vi "3458A Self Calibrate Virtual Channels.vi"(8 "error in":errorcluster, 10 "Ignore GUI, force selfcal (False)":bool, 11 "digitizer session in":T1={"channels"=[], "sync unit"={"VISA"="", "type"=enum."Picotest U6200A"}, "awg unit"={"type"=enum."Agilent 331xxA to 332xxA", "VISA"="", "enable 10MHz ref"=FALSE, "cmi ckd2"={"VISA"="", "clock source"=enum."Auto", "manual ref clk"=FALSE, "ref clock [Hz]"=0.0, "div mode"=enum."Set divisor directly"}, "cmi sync v3"={"VISA"="", "baud rate [bd/s]"=115200, "source"=enum."Auto", "hv range"=enum."1kV", "fsrc is fixed"=FALSE, "fsrc [Hz]"=10000000.0, "freq integ [s]"=1.0, "freq filter"=5, "trig level"=enum."TTL 5V", "chn1 mode"=enum."Source divider", "chn1 level"=enum."Positive 5V", "chn2 mode"=enum."Source divider", "chn2 level"=enum."Positive 5V", "chn2 div"=1, "chn3 mode"=enum."Chn 1 Active", "chn3 level"=enum."Positive 5V", "chn1 div entry"=enum."Calculate nearest divisor from measured fx", "chn1 dev limit [%]"=1.0, "chn1 check dev"=FALSE}, "trigger"={"source"=enum."Immediate", "level [V]"=0.0, "coupling"=enum."DC", "slope"=enum."POS"}}, "sync mode"=enum."MASTER-SLAVE, MASTER clocked by TIMER", "streaming mode"=FALSE, "idn mode"=enum."Auto", "sampling mode"=enum."DCV", "sample memory [B]"=0, "proc setup"={"channel id"=0, "packet size [smpl]"=0, "current timeout [s]"=0.0, "blk2blk timeout [s]"=0.0, "event time"=timestamp(0 s since 1904-01-01), "stop notifier"=refnum, "data queues"=[], "proc refs"=[], "bus semaphore"=refnum}, "sample size [B]"=0, "sample count"=0, "aux data"={"channel id"=0, "valid?"=[], "gain [V]"=[], "timestamp [s]"=[], "Ts [s]"=0.0, "abs timestamp"=timestamp(0 s since 1904-01-01), "t [deg C]"=[], "multiplex timestamp [s]"=-1.0, "only multiplex?"=FALSE, "multiplex smpl offset"=0, "overflow?"=FALSE}, "ranges [V]"=[], "aperture [s]"=0.0, "LEVEL trigger"={"edge"=enum."POS", "level [V]"=0.0, "coupling"=enum."DC"}, "trigger mode"=enum."AUTO", "measure temp.?"=FALSE, "disp mesages"=[], "shared bus?"=FALSE, "disable display?"=FALSE, "aper mode"=enum."Manual", "aper rules"=[], "multiplex"={"cycles"=0, "delay [s]"=0.0, "enabled"=FALSE, "overhead [s]"=1.0, "tot smpls"=0, "sub-rec"=0, "overhead [%]"=0.0, "emulated"=FALSE}, "F8588 lpf"=enum."Off", "F8588 pll"=enum."Off", "F8588 couple"=enum."DC, auto", "fs"={"freq mode"=enum."fs or Ts", "fs [Hz]"=0.0, "fref [Hz]"=0.0, "mul"=0.0, "div"=0.0}} {"awg unit"."cmi sync v3"."chn2 div" min=1 max=100000000 step=1; "awg unit"."cmi sync v3"."fsrc [Hz]" format="%_8p"; "channels"."Range [Vpk]" min=0.0}) -> (0 "error":errorcluster, 3 "digitizer session out":T1={"channels"=[], "sync unit"={"VISA"="", "type"=enum."Picotest U6200A"}, "awg unit"={"type"=enum."Agilent 331xxA to 332xxA", "VISA"="", "enable 10MHz ref"=FALSE, "cmi ckd2"={"VISA"="", "clock source"=enum."Auto", "manual ref clk"=FALSE, "ref clock [Hz]"=0.0, "div mode"=enum."Set divisor directly"}, "cmi sync v3"={"VISA"="", "baud rate [bd/s]"=115200, "source"=enum."Auto", "hv range"=enum."1kV", "fsrc is fixed"=FALSE, "fsrc [Hz]"=10000000.0, "freq integ [s]"=1.0, "freq filter"=5, "trig level"=enum."TTL 5V", "chn1 mode"=enum."Source divider", "chn1 level"=enum."Positive 5V", "chn2 mode"=enum."Source divider", "chn2 level"=enum."Positive 5V", "chn2 div"=1, "chn3 mode"=enum."Chn 1 Active", "chn3 level"=enum."Positive 5V", "chn1 div entry"=enum."Calculate nearest divisor from measured fx", "chn1 dev limit [%]"=1.0, "chn1 check dev"=FALSE}, "trigger"={"source"=enum."Immediate", "level [V]"=0.0, "coupling"=enum."DC", "slope"=enum."POS"}}, "sync mode"=enum."MASTER-SLAVE, MASTER clocked by TIMER", "streaming mode"=FALSE, "idn mode"=enum."Auto", "sampling mode"=enum."DCV", "sample memory [B]"=0, "proc setup"={"channel id"=0, "packet size [smpl]"=0, "current timeout [s]"=0.0, "blk2blk timeout [s]"=0.0, "event time"=timestamp(0 s since 1904-01-01), "stop notifier"=refnum, "data queues"=[], "proc refs"=[], "bus semaphore"=refnum}, "sample size [B]"=0, "sample count"=0, "aux data"={"channel id"=0, "valid?"=[], "gain [V]"=[], "timestamp [s]"=[], "Ts [s]"=0.0, "abs timestamp"=timestamp(0 s since 1904-01-01), "t [deg C]"=[], "multiplex timestamp [s]"=-1.0, "only multiplex?"=FALSE, "multiplex smpl offset"=0, "overflow?"=FALSE}, "ranges [V]"=[], "aperture [s]"=0.0, "LEVEL trigger"={"edge"=enum."POS", "level [V]"=0.0, "coupling"=enum."DC"}, "trigger mode"=enum."AUTO", "measure temp.?"=FALSE, "disp mesages"=[], "shared bus?"=FALSE, "disable display?"=FALSE, "aper mode"=enum."Manual", "aper rules"=[], "multiplex"={"cycles"=0, "delay [s]"=0.0, "enabled"=FALSE, "overhead [s]"=1.0, "tot smpls"=0, "sub-rec"=0, "overhead [%]"=0.0, "emulated"=FALSE}, "F8588 lpf"=enum."Off", "F8588 pll"=enum."Off", "F8588 couple"=enum."DC, auto", "fs"={"freq mode"=enum."fs or Ts", "fs [Hz]"=0.0, "fref [Hz]"=0.0, "mul"=0.0, "div"=0.0}} {"awg unit"."cmi sync v3"."chn2 div" min=1 max=100000000 step=1; "awg unit"."cmi sync v3"."fsrc [Hz]" format="%_8p"; "channels"."Range [Vpk]" min=0.0})   [LabVIEW 2020, in "3458A Virtual Digitizer.lvlib"]
doc: "This VI will allow user to initiate AUTOCAL function on all virtual channels. It will perform DCV calibartion and when the DSDC or DSAC mode is selected it will also perform ACV calibration.\nOptional input 'Ignore GUI' will perform selfcal immediately ignoring GUI buttons, then will close the panel."
uses:
  3458A Virtual Digitizer.lvlib
  3458A Digitizer Session.ctl
  3458A Virtual Channel Config.ctl
  Counter/Counter Session.ctl
  Counter/Counter Type.ctl
  AWG/AWG Session.ctl
  AWG/AWG Type.ctl
  AWG/CMI Clock Divider v2/CMI ckd2 Session.ctl
  AWG/CMI Clock Divider v2/CMI ckd2 Source Mode.ctl
  AWG/CMI Clock Divider v2/CMI ckd2 Divisor Mode.ctl
  AWG/CMI Sync V3/CMI Sync V3 session.ctl
  AWG/CMI Sync V3/Configure/CMI Sync V3 Reference Clock Source.ctl
  AWG/CMI Sync V3/Configure/CMI Sync V3 HV input Range.ctl
  AWG/CMI Sync V3/Configure/CMI Sync V3 Trigger Input Level.ctl
  AWG/CMI Sync V3/Configure/CMI Sync V3 Channel 1 Mode.ctl
  AWG/CMI Sync V3/Configure/CMI Sync V3 Channel Output Levels.ctl
  AWG/CMI Sync V3/Configure/CMI Sync V3 Channel 2 Mode.ctl
  AWG/CMI Sync V3/Configure/CMI Sync V3 Channel 3 Mode.ctl
  AWG/CMI Sync V3/Configure/CMI Sync V3 Channel 1 Divisor Entry Mode.ctl
  adc/ADC Trig Config.ctl
  adc/ADC Trig Mode Source.ctl
  adc/ADC Trig Coupling.ctl
  adc/ADC Trig Slope.ctl
  3458A Sync Mode.ctl
  3458A Idn Mode.ctl
  3458A Digitizing Low Levels/Configure/Sampling Mode.ctl
  3458A Digitizing Process Options.ctl
  3458A Data Packet.ctl
  3458A Aux Record Data.ctl
  3458A Digitizing Low Levels/Configure/Level Setup.ctl
  3458A Digitizing Low Levels/Configure/First Sample Trigger.ctl
  3458A Aperture Selection Mode.ctl
  3458A Multiplexing Config.ctl
  Fluke 8588A/F8588A Low Pass Filter.ctl
  Fluke 8588A/F8588A Phase Lock.ctl
  Fluke 8588A/F8588A Coupling.ctl
  3458A Sampling Rate.ctl
  AWG/AWG Clock Setup Mode.ctl
  3458A Digitizing Low Levels/Action-Status/AutoCal Mode.ctl
  3458A Digitizing Low Levels/3458A Digitizing Low Levels.lvlib
  3458A Basic Driver/3458A Basic Driver.lvlib
  Counter/Counter.lvlib
  AWG/AWG.lvlib
  AWG/CMI Sync V3/CMI Sync Unit V3.lvlib
panel:
  out "instructions":string="1) Disconnect everything from inputs of the DMMs. \n2) Press start to start AUTOCAL.\n3) When done, leave by EXIT.\n4) If it goes wrong, use ABORT to terminate."
  in  "btn abort":bool
  in  "btn exit":bool
  in  "btn start":bool
  out "Status":string
  out "state":i32
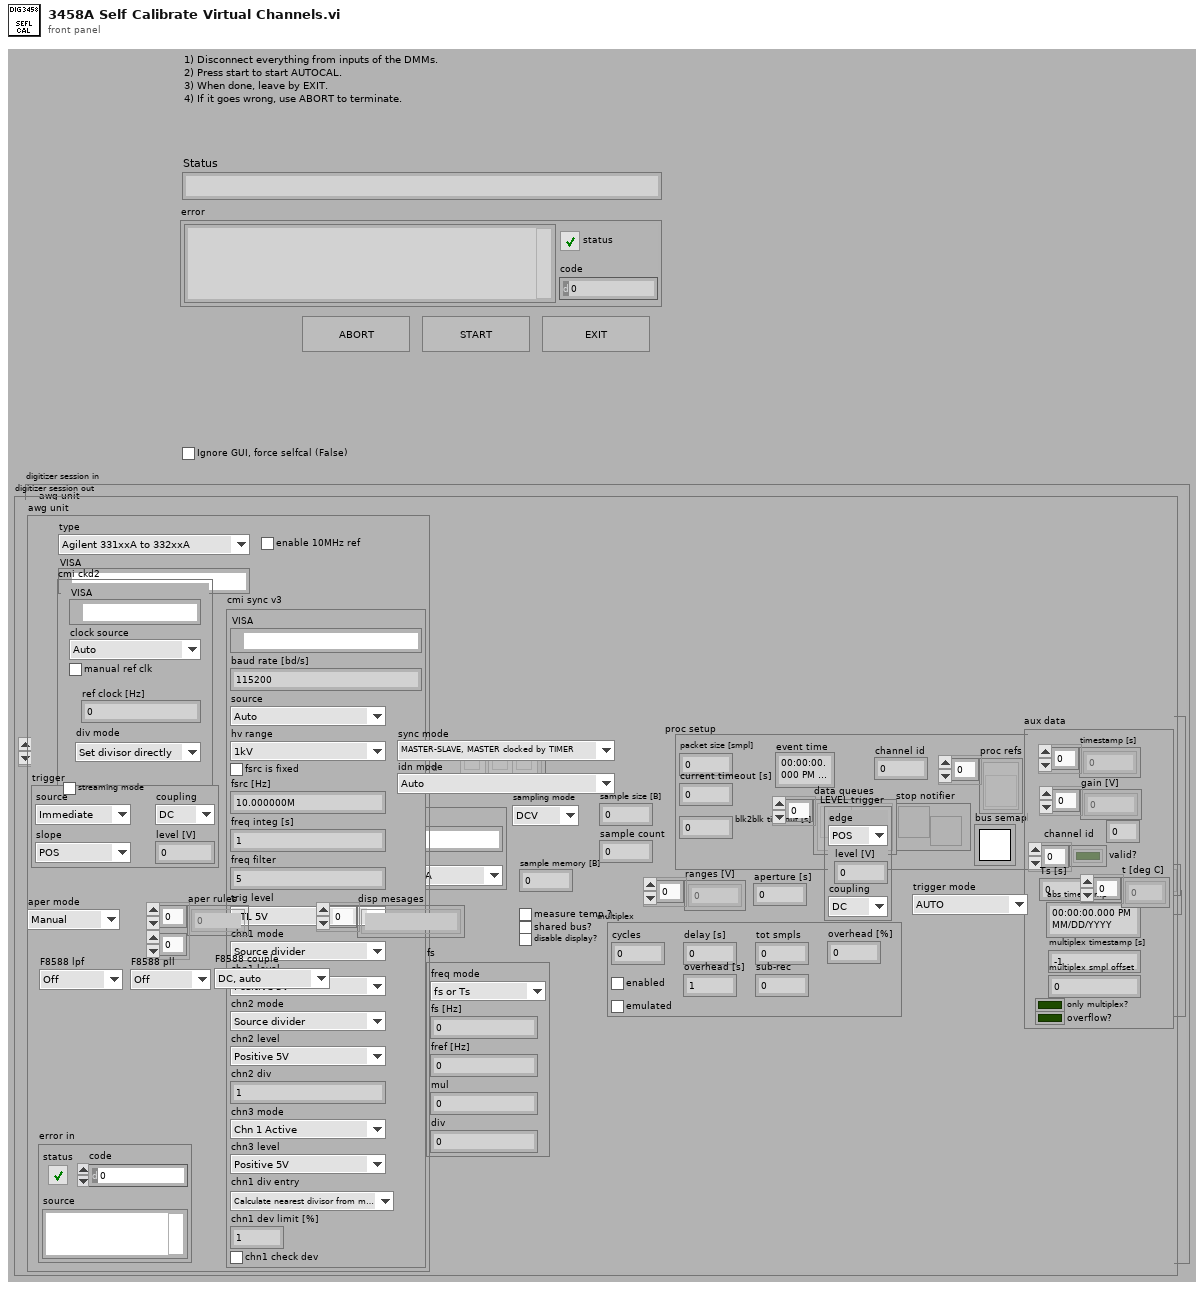
[diagram p1: front panel]
types:
  T1 = typedef "3458A Virtual Digitizer.lvlib/3458A Digitizer Session.ctl" = cluster{"channels":T2[], "sync unit":T3, "awg unit":T5, "sync mode":T23, "streaming mode":bool, "idn mode":T24, "sampling mode":T25, "sample memory [B]":i32, "proc setup":T26, "sample size [B]":i32, "sample count":i32, "aux data":T28, "ranges [V]":dbl[], "aperture [s]":dbl, "LEVEL trigger":T29, "trigger mode":T30, "measure temp.?":bool, "disp mesages":string[], "shared bus?":bool, "disable display?":bool, "aper mode":T31, "aper rules":dbl[][], "multiplex":T32, "F8588 lpf":T33, "F8588 pll":T34, "F8588 couple":T35, "fs":T36}
  T2 = typedef "3458A Virtual Digitizer.lvlib/3458A Virtual Channel Config.ctl" = cluster{"VISA":refnum<visa-resource-name>, "Range [Vpk]":dbl, "btn clr":bool, "btn up":bool, "btn down":bool, "F8588":bool, "F8588 guard":bool}
  T3 = typedef "Counter.lvlib/Counter Session.ctl" = cluster{"VISA":refnum<visa-resource-name>, "type":T4}
  T4 = typedef "Counter.lvlib/Counter Type.ctl" = enum16{"Picotest U6200A", "dummy"}
  T5 = typedef "AWG.lvlib/AWG Session.ctl" = cluster{"type":T6, "VISA":refnum<visa-resource-name>, "enable 10MHz ref":bool, "cmi ckd2":T7, "cmi sync v3":T10, "trigger":T19}
  T6 = typedef "AWG.lvlib/AWG Type.ctl" = enum16{"Agilent 331xxA to 332xxA", "Agilent 335xxA to 336xxA", "Tektronix AFG3101C", "CMI Clock Divider v2", "CMI Sync Unit V3", "dummy"}
  T7 = typedef "AWG.lvlib/CMI ckd2 Session.ctl" = cluster{"VISA":refnum<visa-resource-name>, "clock source":T8, "manual ref clk":bool, "ref clock [Hz]":dbl, "div mode":T9}
  T8 = typedef "AWG.lvlib/CMI ckd2 Source Mode.ctl" = enum16{"Auto", "LF clock", "HF clock", "Internal"}
  T9 = typedef "AWG.lvlib/CMI ckd2 Divisor Mode.ctl" = enum16{"Set divisor directly", "Set divisor by frequency"}
  T10 = typedef "AWG.lvlib/CMI Sync Unit V3.lvlib/CMI Sync V3 session.ctl" = cluster{"VISA":refnum<visa-resource-name>, "baud rate [bd/s]":i32, "source":T11, "hv range":T12, "fsrc is fixed":bool, "fsrc [Hz]":dbl, "freq integ [s]":dbl, "freq filter":i32, "trig level":T13, "chn1 mode":T14, "chn1 level":T15, "chn2 mode":T16, "chn2 level":T15, "chn2 div":i32, "chn3 mode":T17, "chn3 level":T15, "chn1 div entry":T18, "chn1 dev limit [%]":dbl, "chn1 check dev":bool}
  T11 = typedef "AWG.lvlib/CMI Sync Unit V3.lvlib/CMI Sync V3 Reference Clock Source.ctl" = enum16{"Auto", "Internal", "Logic", "Sine", "HV"}
  T12 = typedef "AWG.lvlib/CMI Sync Unit V3.lvlib/CMI Sync V3 HV input Range.ctl" = enum16{"10V", "60V", "250V", "1kV"}
  T13 = typedef "AWG.lvlib/CMI Sync Unit V3.lvlib/CMI Sync V3 Trigger Input Level.ctl" = enum16{"LVCMOS 3V3", "TTL 5V"}
  T14 = typedef "AWG.lvlib/CMI Sync Unit V3.lvlib/CMI Sync V3 Channel 1 Mode.ctl" = enum16{"Source divider", "DDS absolute", "DDS ratio", "DDS ratio M/N"}
  T15 = typedef "AWG.lvlib/CMI Sync Unit V3.lvlib/CMI Sync V3 Channel Output Levels.ctl" = enum16{"Positive 3V3", "Negative 3V3", "Positive 5V", "Negative 5V"}
  T16 = typedef "AWG.lvlib/CMI Sync Unit V3.lvlib/CMI Sync V3 Channel 2 Mode.ctl" = enum16{"Source divider", "Chn 1 divide"}
  T17 = typedef "AWG.lvlib/CMI Sync Unit V3.lvlib/CMI Sync V3 Channel 3 Mode.ctl" = enum16{"Chn 1 Active", "Chn 2 Active", "Chn 1 Trigger", "Chn 2 Trigger", "Gate", "PPS", "10MHz"}
  T18 = typedef "AWG.lvlib/CMI Sync Unit V3.lvlib/CMI Sync V3 Channel 1 Divisor Entry Mode.ctl" = enum16{"Set divisor directly", "Calculate nearest divisor from measured fx"}
  T19 = typedef "ADC Trig Config.ctl" = cluster{"source":T20, "level [V]":dbl, "coupling":T21, "slope":T22}
  T20 = typedef "ADC Trig Mode Source.ctl" = enum16{"Immediate", "External", "Level"}
  T21 = typedef "ADC Trig Coupling.ctl" = enum16{"DC", "AC"}
  T22 = typedef "ADC Trig Slope.ctl" = enum16{"POS", "NEG"}
  T23 = typedef "3458A Virtual Digitizer.lvlib/3458A Sync Mode.ctl" = enum16{"MASTER-SLAVE, MASTER clocked by TIMER", "MASTER-SLAVE, MASTER clocked by AWG", "ALL clocked by AWG", "MASTER-SLAVE, ALL clocked by TIMER", "ALL clocked by AWG with DFLL"}
  T24 = typedef "3458A Virtual Digitizer.lvlib/3458A Idn Mode.ctl" = enum16{"Auto", "Sequential (chn A, chn B, ...)", "From calibration string"}
  T25 = typedef "3458A Virtual Digitizer.lvlib/3458A Digitizing Low Levels.lvlib/Sampling Mode.ctl" = enum16{"DCV", "DSDC", "DSAC"}
  T26 = typedef "3458A Virtual Digitizer.lvlib/3458A Digitizing Process Options.ctl" = cluster{"channel id":i32, "packet size [smpl]":i32, "current timeout [s]":dbl, "blk2blk timeout [s]":dbl, "event time":timestamp, "stop notifier":refnum<notifier>, "data queues":refnum<queue>[], "proc refs":refnum<vi>[], "bus semaphore":T27}
  T27 = typedef "Semaphore RefNum" = refnum<k1>
  T28 = typedef "3458A Virtual Digitizer.lvlib/3458A Aux Record Data.ctl" = cluster{"channel id":i32, "valid?":bool[], "gain [V]":dbl[], "timestamp [s]":dbl[], "Ts [s]":dbl, "abs timestamp":timestamp, "t [deg C]":dbl[], "multiplex timestamp [s]":dbl, "only multiplex?":bool, "multiplex smpl offset":i64, "overflow?":bool}
  T29 = typedef "3458A Virtual Digitizer.lvlib/3458A Digitizing Low Levels.lvlib/Level Setup.ctl" = cluster{"edge":enum16{"POS", "NEG"}, "level [V]":dbl, "coupling":enum16{"DC", "AC"}}
  T30 = typedef "3458A Virtual Digitizer.lvlib/3458A Digitizing Low Levels.lvlib/First Sample Trigger.ctl" = enum16{"AUTO", "EXT", "SYN", "SGL", "HOLD", "LEVEL"}
  T31 = typedef "3458A Virtual Digitizer.lvlib/3458A Aperture Selection Mode.ctl" = enum16{"Manual", "Maximum", "Table"}
  T32 = typedef "3458A Virtual Digitizer.lvlib/3458A Multiplexing Config.ctl" = cluster{"cycles":i32, "delay [s]":dbl, "enabled":bool, "overhead [s]":dbl, "tot smpls":i64, "sub-rec":i32, "overhead [%]":dbl, "emulated":bool}
  T33 = typedef "F8588A Low Pass Filter.ctl" = enum16{"Off", "100 kHz", "3 MHz"}
  T34 = typedef "F8588A Phase Lock.ctl" = enum16{"Off", "1 MHz", "10 MHz"}
  T35 = typedef "F8588A Coupling.ctl" = enum16{"AC, 1 MOhm", "AC, 10 MOhm", "DC, 1 MOhm", "DC, 10 MOhm", "DC, auto"}
  T36 = typedef "3458A Virtual Digitizer.lvlib/3458A Sampling Rate.ctl" = cluster{"freq mode":T37, "fs [Hz]":dbl, "fref [Hz]":dbl, "mul":dbl, "div":dbl}
  T37 = typedef "AWG.lvlib/AWG Clock Setup Mode.ctl" = enum16{"fs or Ts", "fs or Ts with fref", "fref/N", "fref*M/N", "fref*Ratio"}
  T38 = typedef "3458A Virtual Digitizer.lvlib/3458A Digitizing Low Levels.lvlib/AutoCal Mode.ctl" = enum16{"ALL", "DCV", "AC", "OHMS"}
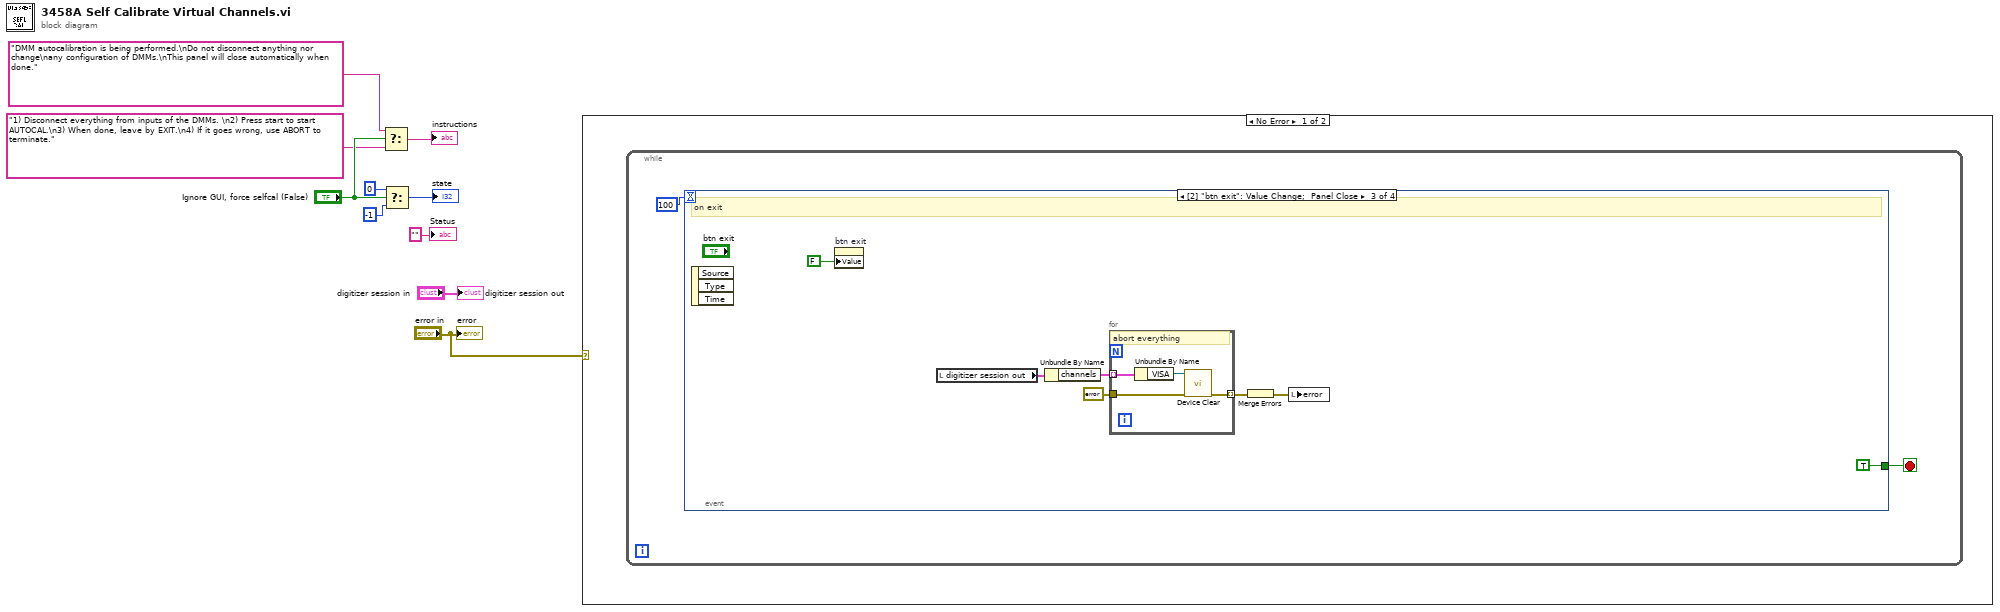
[diagram p0: block diagram]
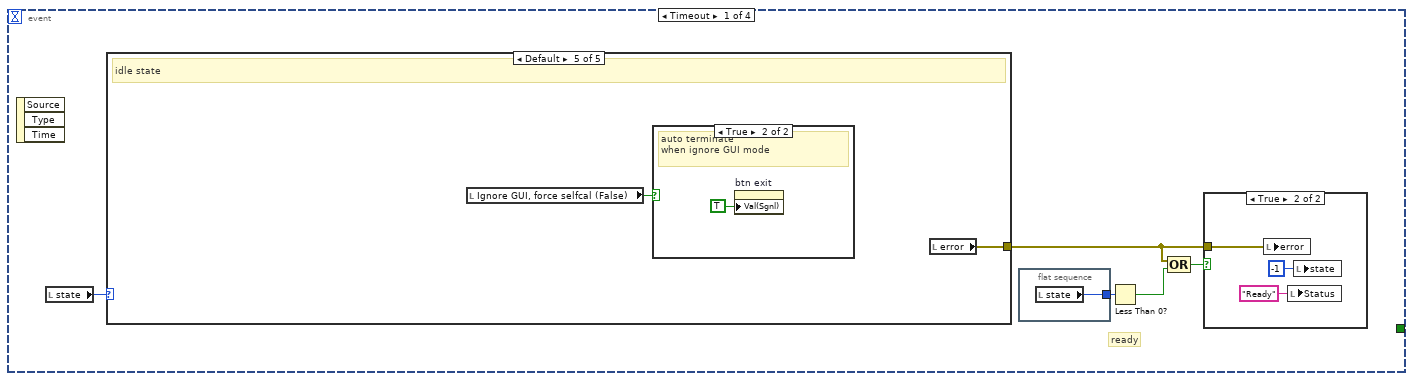
[diagram p2: hidden frame]
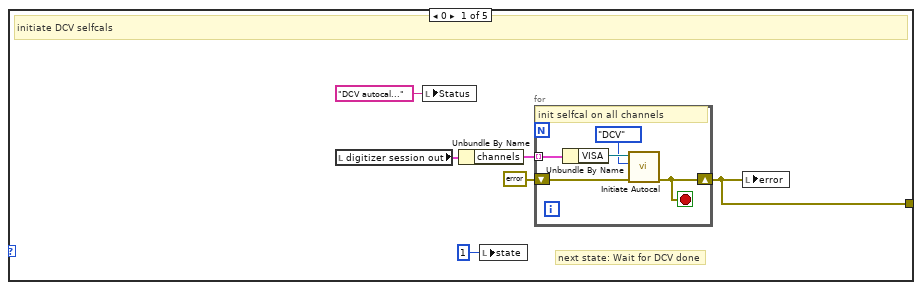
[diagram p4: hidden frame]
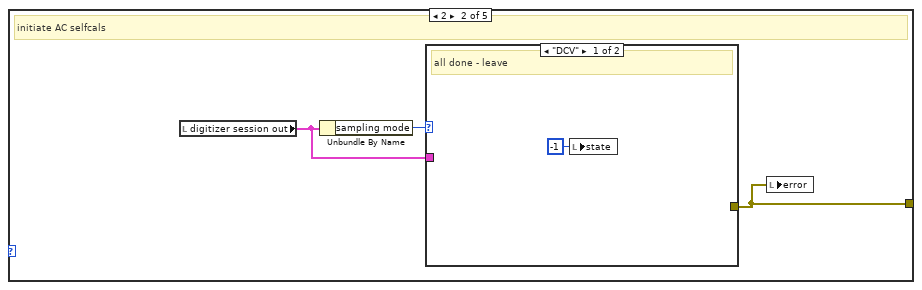
[diagram p5: hidden frame]
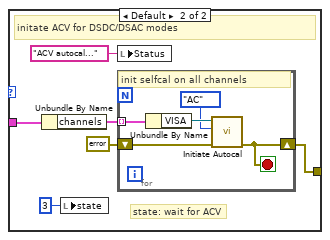
[diagram p6: hidden frame]
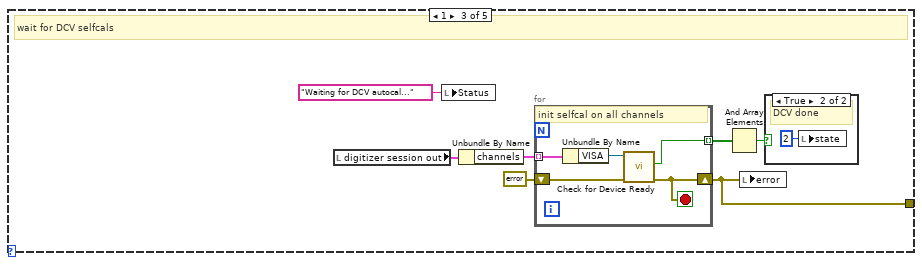
[diagram p7: hidden frame]
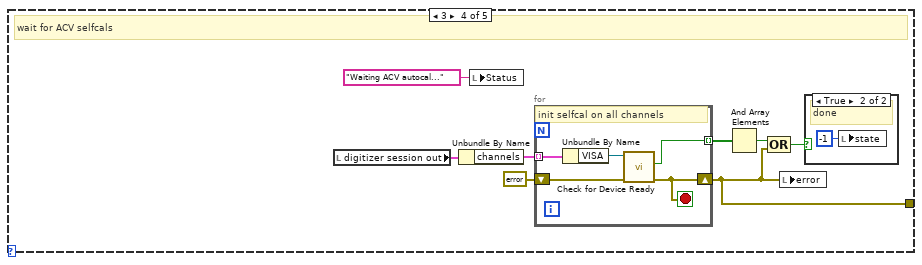
[diagram p9: hidden frame]
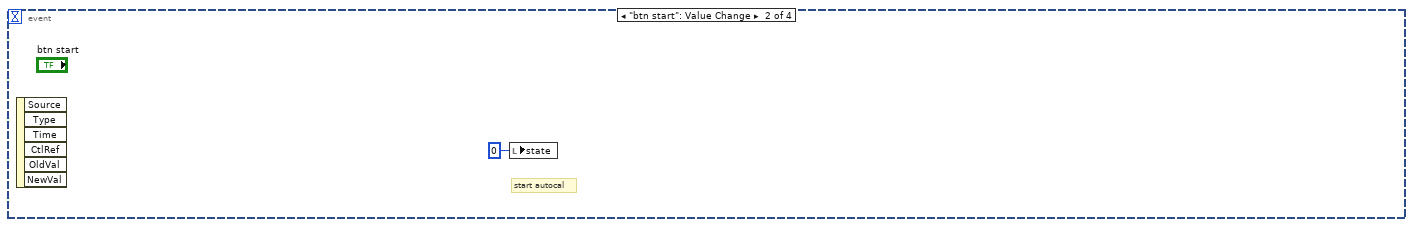
[diagram p12: hidden frame]
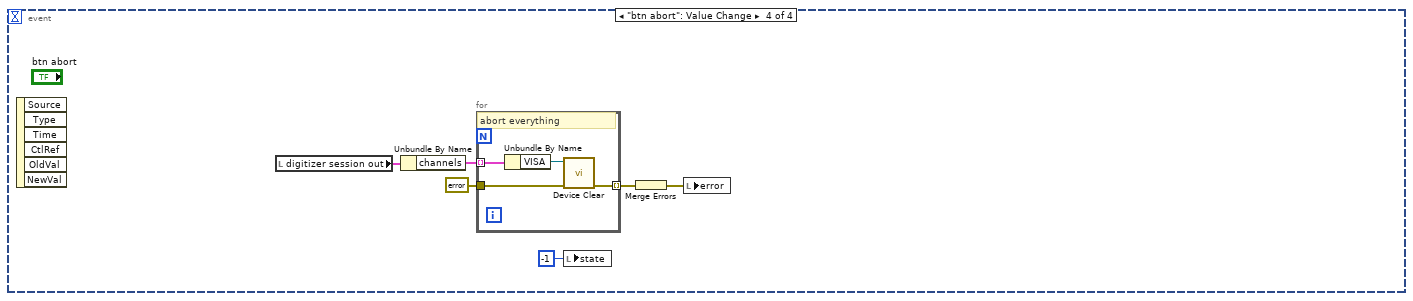
[diagram p13: hidden frame]
diagram:
  n1 = Select(t="DMM autocalibration is being performed.\nDo not disconnect anything nor change\nany configuration of DMMs.\nThis panel will close automatically when done." ("Status"), s="Ignore GUI, force selfcal (False)", f="1) Disconnect everything from inputs of the DMMs. \n2) Press start to start AUTOCAL.\n3) When done, leave by EXIT.\n4) If it goes wrong, use ABORT to terminate." ("Status")) -> (s? t:f=→"instructions":string)
  n2 = Select(t=0, s="Ignore GUI, force selfcal (False)", f=-1 ("state")) -> (s? t:f=→"state":i32)
  n3 = case shown="No Error" "error in" {
    frame No Error {
      n4 = while {
        stop <- w11 stop-if-true
        n5 = event shown="[2] \"btn exit\": Value Change;  Panel Close" {
          selector: _ -> [_ _ _ _]
          dyn-events: _ -> [_ _ _ _]
          timeout: 100 -> [_ _ _ _]
          tunnel: [_ _ TRUE _] -> w11
          event Timeout {
            # "ready"
            n6 = event-data() -> ()  [unwired: 1 in, 3 out]
            n7 = local read "state"() -> (w17:i32)
            n8 = case shown="Default" w17 {
              tunnel: [w22 w35 w52 w61 w76] -> w15
              frame 0 {
                # "next state: Wait for DCV done"
                # "initiate DCV selfcals"
                n9 = local read "digitizer session out"() -> (w24:T1)
                n10 = local write "Status"("DCV autocal..." ("Status")) -> ()
                n11 = Unbundle By Name(w24) -> ("channels"=w27:T2[])
                n12 = local write "state"(1) -> ()
                n13 = for {
                  tunnel: w27 -> [w30] mode=indexing
                  shift-right: [w29] -> w22
                  shift-left: errorcluster {"status"=FALSE, "code"=0, "source"=""} ("error out") -> [w32]
                  stop <- w29 stop-if-true
                  # "init selfcal on all channels"
                  n14 = Unbundle By Name(w30) -> ("VISA"=w31:refnum<visa-resource-name>)
                  n15 = call "Initiate Autocal.vi"("error in"=w32, "mode (ALL)"=AutoCal_Mode."DCV", "VISA resource in"=w31) -> ("error out"=w29:errorcluster)  [unwired: 7 in, 1 out]
                }
                n16 = local write "error"(w22) -> ()
              }
              frame 2 {
                # "initiate AC selfcals"
                n17 = local read "digitizer session out"() -> (w34:T1)
                n18 = Unbundle By Name(w34) -> ("sampling mode"=w33:T25)
                n19 = case shown="\"DCV\"" w33 {
                  tunnel: [_ w40] -> w35
                  tunnel: w34 -> [_ w39]
                  frame "DCV" {
                    # "all done - leave"
                    n20 = local write "state"(-1) -> ()
                  }
                  frame Default {
                    # "state: wait for ACV"
                    # "initate ACV for DSDC/DSAC modes"
                    n21 = Unbundle By Name(w39) -> ("channels"=w42:T2[])
                    n22 = local write "state"(3 ("state")) -> ()
                    n23 = local write "Status"("ACV autocal..." ("Status")) -> ()
                    n24 = for {
                      tunnel: w42 -> [w45] mode=indexing
                      shift-right: [w44] -> w40
                      shift-left: errorcluster {"status"=FALSE, "code"=0, "source"=""} ("error out") -> [w47]
                      stop <- w44 stop-if-true
                      # "init selfcal on all channels"
                      n25 = Unbundle By Name(w45) -> ("VISA"=w46:refnum<visa-resource-name>)
                      n26 = call "Initiate Autocal.vi"("error in"=w47, "mode (ALL)"=AutoCal_Mode."AC", "VISA resource in"=w46) -> ("error out"=w44:errorcluster)  [unwired: 7 in, 1 out]
                    }
                  }
                }
                n27 = local write "error"(w35) -> ()
              }
              frame 1 {
                # "wait for DCV selfcals"
                n28 = local read "digitizer session out"() -> (w49:T1)
                n29 = local write "Status"("Waiting for DCV autocal..." ("Status")) -> ()
                n30 = Unbundle By Name(w49) -> ("channels"=w54:T2[])
                n31 = for {
                  tunnel: w54 -> [w58] mode=indexing
                  shift-right: [w57] -> w52
                  shift-left: errorcluster {"status"=FALSE, "code"=0, "source"=""} ("error out") -> [w60]
                  tunnel: [w56] -> w51 mode=indexing
                  stop <- w57 stop-if-true
                  # "init selfcal on all channels"
                  n32 = Unbundle By Name(w58) -> ("VISA"=w59:refnum<visa-resource-name>)
                  n33 = call "Check for Device Ready.vi"("error in"=w60, "VISA resource in"=w59) -> ("error out"=w57:errorcluster, "device ready?"=w56:bool)  [unwired: 7 in, 1 out]
                }
                n34 = And Array Elements(Boolean array=w51) -> (logical AND=w50:bool)
                n35 = local write "error"(w52) -> ()
                n36 = case shown="True" w50 {
                  frame False {
                  }
                  frame True {
                    # "DCV done"
                    n37 = local write "state"(2 ("state")) -> ()
                  }
                }
              }
              frame 3 {
                # "wait for ACV selfcals"
                n38 = local read "digitizer session out"() -> (w65:T1)
                n39 = Unbundle By Name(w65) -> ("channels"=w68:T2[])
                n40 = local write "Status"("Waiting ACV autocal..." ("Status")) -> ()
                n41 = for {
                  tunnel: w68 -> [w72] mode=indexing
                  shift-right: [w71] -> w61
                  shift-left: errorcluster {"status"=FALSE, "code"=0, "source"=""} ("error out") -> [w74]
                  tunnel: [w70] -> w66 mode=indexing
                  stop <- w71 stop-if-true
                  # "init selfcal on all channels"
                  n42 = Unbundle By Name(w72) -> ("VISA"=w73:refnum<visa-resource-name>)
                  n43 = call "Check for Device Ready.vi"("error in"=w74, "VISA resource in"=w73) -> ("error out"=w71:errorcluster, "device ready?"=w70:bool)  [unwired: 7 in, 1 out]
                }
                n44 = And Array Elements(Boolean array=w66) -> (logical AND=w63:bool)
                n45 = Compound Arithmetic op=OR(w63, w61) -> (w62:bool)
                n46 = local write "error"(w61) -> ()
                n47 = case shown="True" w62 {
                  frame False {
                  }
                  frame True {
                    # "done"
                    n48 = local write "state"(-1 ("state")) -> ()
                  }
                }
              }
              frame Default {
                # "idle state"
                n49 = local read "Ignore GUI, force selfcal (False)"() -> (w75:bool)
                n50 = case shown="True" w75 {
                  frame False {
                  }
                  frame True {
                    # "auto terminate\nwhen ignore GUI mode"
                    n51 = property on="btn exit" class="Bool (strict)"("Val(Sgnl)"=TRUE) -> ()  [unwired: 2 in, 2 out]
                  }
                }
                n52 = local read "error"() -> (w76:errorcluster)
              }
            }
            n53 = flat-sequence {
              tunnel: [w21] -> w16
              frame #0 {
                n54 = local read "state"() -> (w21:i32)
              }
            }
            n55 = Less Than 0?(x=w16) -> (x < 0?=w14:bool)
            n56 = Compound Arithmetic op=OR(w15, w14) -> (w13:bool)
            n57 = case shown="True" w13 {
              tunnel: w15 -> [_ w19]
              frame False {
              }
              frame True {
                n58 = local write "error"(w19) -> ()
                n59 = local write "Status"("Ready" ("Status")) -> ()
                n60 = local write "state"(-1 ("state")) -> ()
              }
            }
          }
          event "btn start": Value Change {
            # "start autocal"
            n61 = event-data() -> ()  [unwired: 1 in, 6 out]
            n62 = local write "state"(0 ("state")) -> ()
          }
          event "btn exit": Value Change; Panel Close {
            # "on exit"
            n63 = event-data() -> ()  [unwired: 1 in, 3 out]
            n64 = property on="btn exit" class="Bool (strict)"("Value"=FALSE) -> ()  [unwired: 2 in, 2 out]
            n65 = local read "digitizer session out"() -> (w83:T1)
            n66 = Unbundle By Name(w83) -> ("channels"=w85:T2[])
            n67 = for {
              tunnel: w85 -> [w89] mode=indexing
              tunnel: errorcluster {"status"=FALSE, "code"=0, "source"=""} ("error out") -> [w88]
              tunnel: [w86] -> w82 mode=indexing
              # "abort everything"
              n68 = Unbundle By Name(w89) -> ("VISA"=w87:refnum<visa-resource-name>)
              n69 = call "Device Clear.vi"("error in(no error)"=w88, "VISA Resource Name"=w87) -> ("error out"=w86:errorcluster)  [unwired: 8 in, 1 out]
            }
            n70 = Merge Errors(w82) -> (w81:errorcluster)
            n71 = local write "error"(w81) -> ()
          }
          event "btn abort": Value Change {
            n72 = event-data() -> ()  [unwired: 1 in, 6 out]
            n73 = local read "digitizer session out"() -> (w93:T1)
            n74 = Unbundle By Name(w93) -> ("channels"=w95:T2[])
            n75 = for {
              tunnel: w95 -> [w99] mode=indexing
              tunnel: errorcluster {"status"=FALSE, "code"=0, "source"=""} ("error out") -> [w98]
              tunnel: [w96] -> w92 mode=indexing
              # "abort everything"
              n76 = Unbundle By Name(w99) -> ("VISA"=w97:refnum<visa-resource-name>)
              n77 = call "Device Clear.vi"("error in(no error)"=w98, "VISA Resource Name"=w97) -> ("error out"=w96:errorcluster)  [unwired: 8 in, 1 out]
            }
            n78 = local write "state"(-1 ("state")) -> ()
            n79 = Merge Errors(w92) -> (w91:errorcluster)
            n80 = local write "error"(w91) -> ()
          }
        }
      }
    }
    frame Error {
    }
  }
  "digitizer session out" <- "digitizer session in"
  "error" <- "error in"
  "Status" <- "" ("Status")
